vi "Calibrate.vi"(3 "Deviceindex":i32) -> (0 "Calib Error":bool, 1 "Status":string)   [LabVIEW 2019]
uses:
  phlib.dll
panel:
  out "Returncode":i32
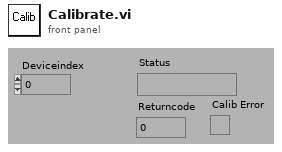
[diagram p1: front panel]
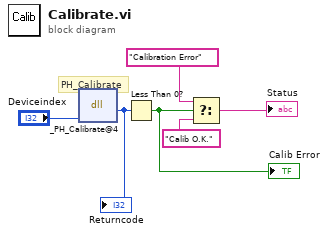
[diagram p0: block diagram]
diagram:
  # "PH_Calibrate"
  n1 = dll-call lib="phlib.dll" fn="_PH_Calibrate@4"("devidx"="Deviceindex") -> (w4:i32)  [unwired: 4 in, 2 out]
  "Returncode" <- w4
  n2 = Less Than 0?(x=w4) -> (x < 0?=w2:bool)
  "Calib Error" <- w2
  n3 = Select(t="Calibration Error", s=w2, f="Calib O.K.") -> (s? t:f=→"Status":string)
